vi "图片多色保存2.vi"() -> ()   [LabVIEW 2018]
uses:
  <vilib>/vision/NI_Vision_Development_Module.lvlib
panel:
  out "Image":T1(plugin-control)
  in  "停止":bool
  in  "Image Type":T2 items=["Grayscale (U8)", "Grayscale (I16)", "Grayscale (SGL)", "Complex (CSG)", "RGB (U32)", "HSL (U32)", "RGB (U64)", "Grayscale (U16)"]
  in  "File Path":path
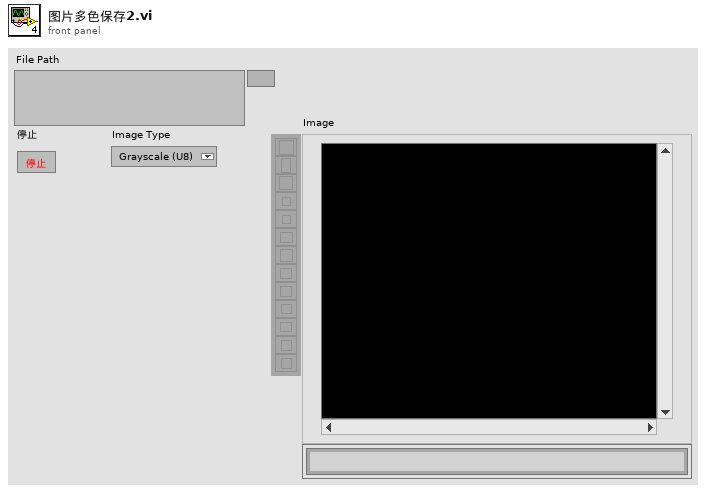
[diagram p1: front panel]
types:
  T1 = typedef "IMAQ Image.ctl" = refnum<image>
  T2 = typedef "Image Type" = u32
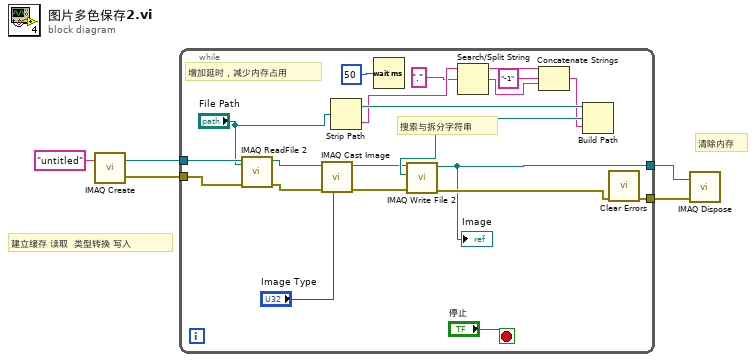
[diagram p0: block diagram]
diagram:
  # "清除内存"
  # "建立缓存 读取  类型转换 写入"
  n1 = call "IMAQ Create"("Image Name"="untitled") -> ("New Image"=w5:T1, "error out"=w4:errorcluster)  [unwired: 4 in]
  n2 = while {
    tunnel: w5 -> [w26]
    tunnel: w4 -> [w24]
    tunnel: [w7] -> w2
    tunnel: [w6] -> w1
    stop <- "停止" stop-if-true
    # "搜索与拆分字符串"
    # "增加延时，减少内存占用"
    n3 = call "IMAQ ReadFile 2"("File Path"="File Path", "error in (no error)"=w24, "Image"=w26) -> ("error out"=w23:errorcluster, "Image Out"=w25:T1)  [unwired: 4 in, 3 out]
    n4 = call "IMAQ Cast Image"("Image Type"="Image Type", "error in (no error)"=w23, "Image Src"=w25) -> ("error out"=w22:errorcluster, "Image Dst Out"=w16:T1)  [unwired: 7 in]
    n5 = Strip Path(path="File Path") -> (stripped path=w19:path, name=w14:string)
    n6 = Wait (ms)(milliseconds to wait=u32 50 ("等待时间（毫秒）")) -> ()  [unwired: 1 out]
    n7 = Search/Split String(string=w14, search string/char (-)="." ("正则表达式")) -> (substring before match=w12:string, match + rest of string=w8:string)  [unwired: 1 in, 1 out]
    n8 = Concatenate Strings(w12, "-1" ("字符串"), w8) -> (w10:string)
    n9 = Build Path(base path=w19, name or relative path=w10) -> (appended path=w18:path)
    n10 = call-poly "IMAQ Write File 2"("error in (no error)"=w22, "File Path"=w18, "Image"=w16) -> ("error out"=w9:errorcluster, "Image Out (duplicate)"=w6:T1)  [unwired: 7 in]
    "Image" <- w6
    n11 = call <vilib>:"Clear Errors.vi"("error in (no error)"=w9) -> ("error out"=w7:errorcluster)  [unwired: 5 in, 1 out]
  }
  n12 = call "IMAQ Dispose"("Image"=w1, "error in (no error)"=w2) -> ()  [unwired: 4 in, 1 out]
